vi "MAIN Printer Reconnect.vi"(8 "error in (no error)":errorcluster, 11 "Domino Laser module Class in":refnum<class "Domino Laser module Class.lvclass">) -> (0 "error out":errorcluster, 3 "Domino Laser module Class out":refnum<class "Domino Laser module Class.lvclass">)   [LabVIEW 2015, in "Domino LM.lvlib" / "Domino Laser module Class.lvclass"]
uses:
  CTRLS/Domino Laser module Class.lvclass
  CTRLS/Domino Laser module Class.lvclass/Domino Laser module Class.ctl
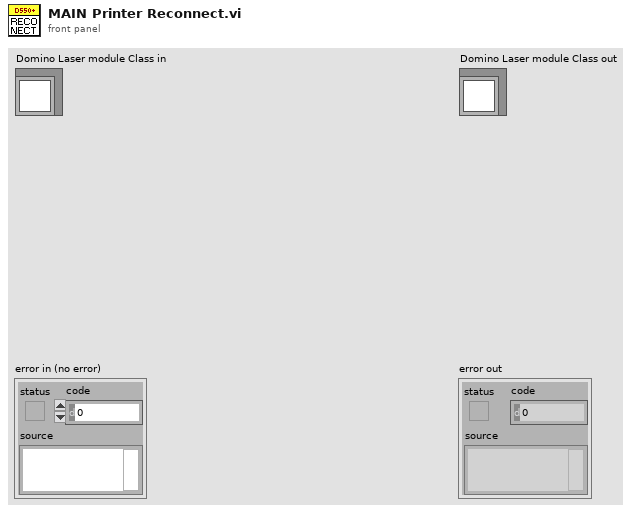
[diagram p1: front panel]
types:
  T1 = enum16{"Standard", "Buffered", "CRLF", "Immediate"}
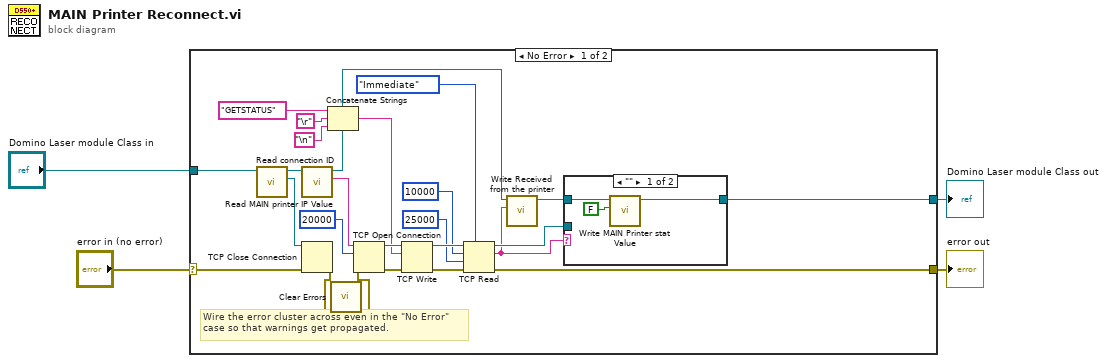
[diagram p0: block diagram]
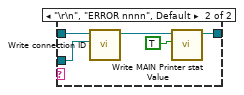
[diagram p2: hidden frame]
diagram:
  n1 = case shown="No Error" "error in (no error)" {
    selector: "error in (no error)" -> [w10 w39]
    tunnel: [w9 w39] -> w3
    tunnel: [w7 w38] -> w1
    tunnel: "Domino Laser module Class in" -> [w13 w38]
    frame No Error {
      # "Wire the error cluster across even in the \"No Error\"\ncase so that warnings get propagated."
      n2 = call "Read connection ID.vi"("Domino Laser module Class in"=w13) -> ("connection ID"=w11:refnum<k5>, "Domino Laser module Class out"=w12:refnum<class "Domino Laser module Class.lvclass">)  [unwired: 8 in, 1 out]
      n3 = call "Read MAIN printer IP Value.vi"("Domino Laser module Class in"=w12) -> ("printer IP value"=w14:string, "Domino Laser module Class out"=w8:refnum<class "Domino Laser module Class.lvclass">)  [unwired: 8 in, 1 out]
      n4 = TCP Close Connection(connection ID=w11, error in (no error)=w10) -> (error out=w6:errorcluster)  [unwired: 1 in, 1 out]
      n5 = Concatenate Strings("GETSTATUS" ("data in"), "\r", "\n") -> (w19:string)
      n6 = call <vilib>:"Clear Errors.vi"("error in (no error)"=w6) -> ("error out"=w5:errorcluster)  [unwired: 5 in, 1 out]
      n7 = TCP Open Connection(address=w14, remote port or service name=u16 20000, error in (no error)=w5) -> (connection ID=w26:refnum<k5>, error out=w27:errorcluster)  [unwired: 2 in]
      n8 = TCP Write(connection ID=w26, data in=w19, error in (no error)=w27) -> (connection ID out=w25:refnum<k5>, error out=w24:errorcluster)  [unwired: 1 in, 1 out]
      n9 = TCP Read(connection ID=w25, bytes to read=10000, error in (no error)=w24, 7:T1."Immediate" ("mode (standard)"), 9:25000 ("timeout ms (25000)")) -> (connection ID out=w23:refnum<k5>, data out=w15:string, error out=w9:errorcluster)
      n10 = call "Write Received from the printer.vi"("Received from the printer"=w15, "Domino Laser module Class in"=w8) -> ("Domino Laser module Class out"=w16:refnum<class "Domino Laser module Class.lvclass">)  [unwired: 8 in, 1 out]
      n11 = case shown="\"\"" w15 {
        tunnel: w16 -> [w32 w37]
        tunnel: [w31 w35] -> w7
        tunnel: w23 -> [_ w36]
        frame "" {
          n12 = call "Write MAIN Printer stat Value.vi"("Printer MIAN status"=FALSE ("Printer status"), "Domino Laser module Class in"=w32) -> ("Domino Laser module Class out"=w31:refnum<class "Domino Laser module Class.lvclass">)  [unwired: 8 in, 1 out]
        }
        frame "\r\n", "ERROR nnnn", Default {
          n13 = call "Write connection ID.vi"("connection ID"=w36, "Domino Laser module Class in"=w37) -> ("Domino Laser module Class out"=w34:refnum<class "Domino Laser module Class.lvclass">)  [unwired: 8 in, 1 out]
          n14 = call "Write MAIN Printer stat Value.vi"("Printer MIAN status"=TRUE ("Printer status"), "Domino Laser module Class in"=w34) -> ("Domino Laser module Class out"=w35:refnum<class "Domino Laser module Class.lvclass">)  [unwired: 8 in, 1 out]
        }
      }
    }
    frame Error {
    }
  }
  "error out" <- w3
  "Domino Laser module Class out" <- w1
